vi "getGraphsInfo.vi"() -> (1 "noOFCurvesInEachGraph":u32[](array[numeric]), 2 "curveNames":string[][](array[string]), 3 "units":string[](array[string]))   [LabVIEW 2024]
uses:
  OVA32.dll
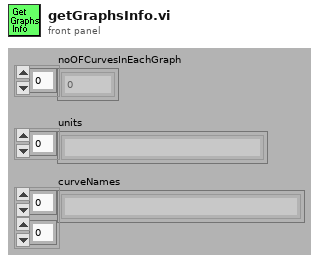
[diagram p1: front panel]
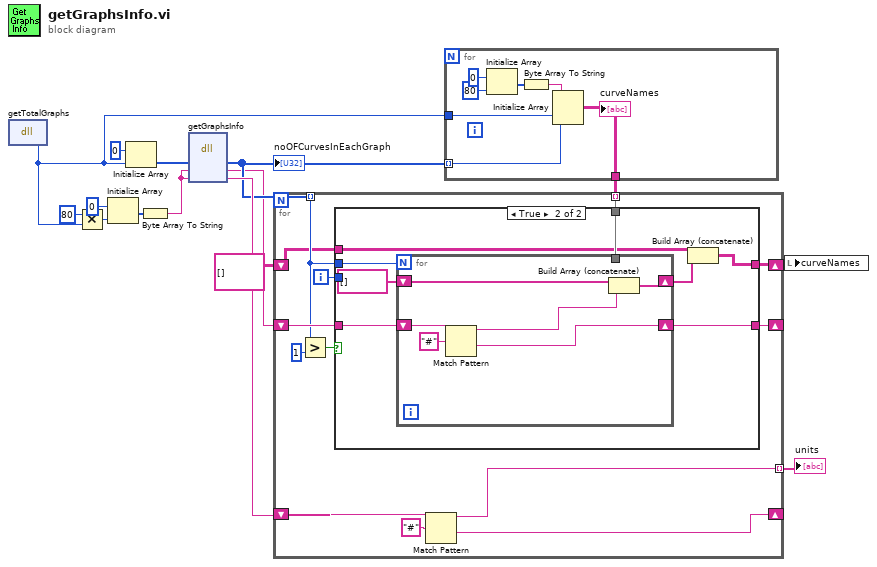
[diagram p0: block diagram]
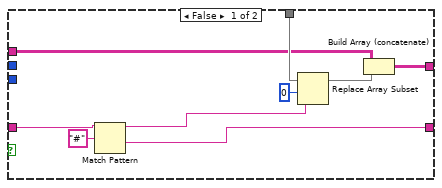
[diagram p2: hidden frame]
diagram:
  n1 = dll-call lib="OVA32.dll" fn="getTotalGraphs"() -> (w5:i32)  [unwired: 3 in, 2 out]
  n2 = Multiply(x=80, y=w5) -> (x*y=w13:i32)
  n3 = Initialize Array(u8 0 ("element"), w13) -> (w12:u8[])
  n4 = Initialize Array(u16 0 ("Element Data"), w5) -> (w15:u16[])
  n5 = Byte Array To String(unsigned byte array=w12) -> (string=w10:string)
  n6 = dll-call lib="OVA32.dll" fn="getGraphsInfo"("noOFCurvesInEachGraph"=w15, "graphTitle"=w10, "graphUnits"=w10) -> ("noOFCurvesInEachGraph"=w8:u16[], "graphTitle"=w6:string, "graphUnits"=w9:string)  [unwired: 4 in, 2 out]
  "noOFCurvesInEachGraph" <- w8
  n7 = for {
    tunnel: w5 -> [w22]
    tunnel: w8 -> [w21] mode=indexing
    tunnel: [w16] -> w4
    n8 = Initialize Array(u16 0 ("Element Data"), 80 ("Dimension Size")) -> (w18:u16[])
    n9 = Byte Array To String(unsigned byte array=w18) -> (string=w17:string)
    n10 = Initialize Array(w17, w22, w21) -> (w16:string[][])
    "curveNames" <- w16
  }
  n11 = for {
    shift-right: [w32] -> _
    shift-left: w6 -> [w33]
    shift-right: [w31] -> _
    shift-left: w9 -> [w35]
    tunnel: w8 -> [w27] mode=indexing
    tunnel: [w34] -> w7 mode=indexing
    tunnel: w4 -> [w25] mode=indexing
    shift-right: [w23] -> w3
    shift-left: string[][] [] -> [w24]
    i -> [w26]
    n12 = Greater?(x=w27, y=u16 1) -> (0:w28:bool)
    n13 = case shown="True" w28 {
      tunnel: w33 -> [w44 w52]
      tunnel: [w43 w51] -> w32
      tunnel: w27 -> [_ w46]
      tunnel: w26 -> [_ _]
      tunnel: w25 -> [w41 w50]
      tunnel: w24 -> [w37 w49]
      tunnel: [w36 w48] -> w23
      frame False {
        n14 = Match Pattern(string=w44, regular expression="#" ("search string/char (-)")) -> (before substring=w39:string, after substring=w43:string)  [unwired: 1 in, 2 out]
        n15 = Replace Array Subset(array=w41, new element=w39, index=0 ("Index")) -> (w38:string[])
        n16 = Build Array (concatenate)(w37, w38) -> (w36:string[][])
      }
      frame True {
        n17 = for {
          N: w46 -> [_]
          shift-right: [w57] -> w51
          shift-left: w52 -> [w56]
          tunnel: w50 -> [_]
          shift-right: [w54] -> w47
          shift-left: string[] [] -> [w53]
          n18 = Match Pattern(string=w56, regular expression="#" ("search string/char (-)")) -> (before substring=w55:string, after substring=w57:string)  [unwired: 1 in, 2 out]
          n19 = Build Array (concatenate)(w53, w55) -> (w54:string[])
        }
        n20 = Build Array (concatenate)(w49, w47) -> (w48:string[][])
      }
    }
    n21 = Match Pattern(string=w35, regular expression="#") -> (before substring=w34:string, after substring=w31:string)  [unwired: 1 in, 2 out]
  }
  "units" <- w7
  n22 = local write "curveNames"(w3) -> ()
